vi "Main_Dev.vi"() -> ()   [LabVIEW 2020]
uses:
  <vilib>/Utility/file.llb/Read Delimited Spreadsheet (I64).vi
  <vilib>/Instr/_visa.llb/VISA Configure Serial Port (Serial Instr).vi
panel:
  out "Next MPH":u16
  out "Next Duration":u16
  out "Next Inc":u16
  out "PD READ 2":u8
  out "PD READ":u8
  out "INC READ":u8
  out "INC READ 2":u8
  out "MPH READ":u8
  out "MPH READ 2":u8
  out "dwell":u16[](array[numeric])
  out "incline":u16[](array[numeric])
  out "time":u16[](array[numeric])
  out "speed":u16[](array[numeric])
  out "selected path":path
  out "input lines":i32
  in  "TestScript":path=path "C:/LabView Computer Backup SEAL2788/DonP_TRM500/FootTimeInc.txt"
  out "refnum out":refnum<file>
  out "read buffer":string
  out "Target Changed":bool
  in  "stop":bool
  in  "Serial Port":refnum<visa-resource-name>="COM8"
  out "FootPath":path
  out "FootPathRef":refnum<file>
  out "stopping":bool
  out "Target MPH":u16 max=12 step=1
  out "step":i32
  out "ESTOP":bool
  out "ESTOP2":bool
  out "INC":u16 max=12 step=1
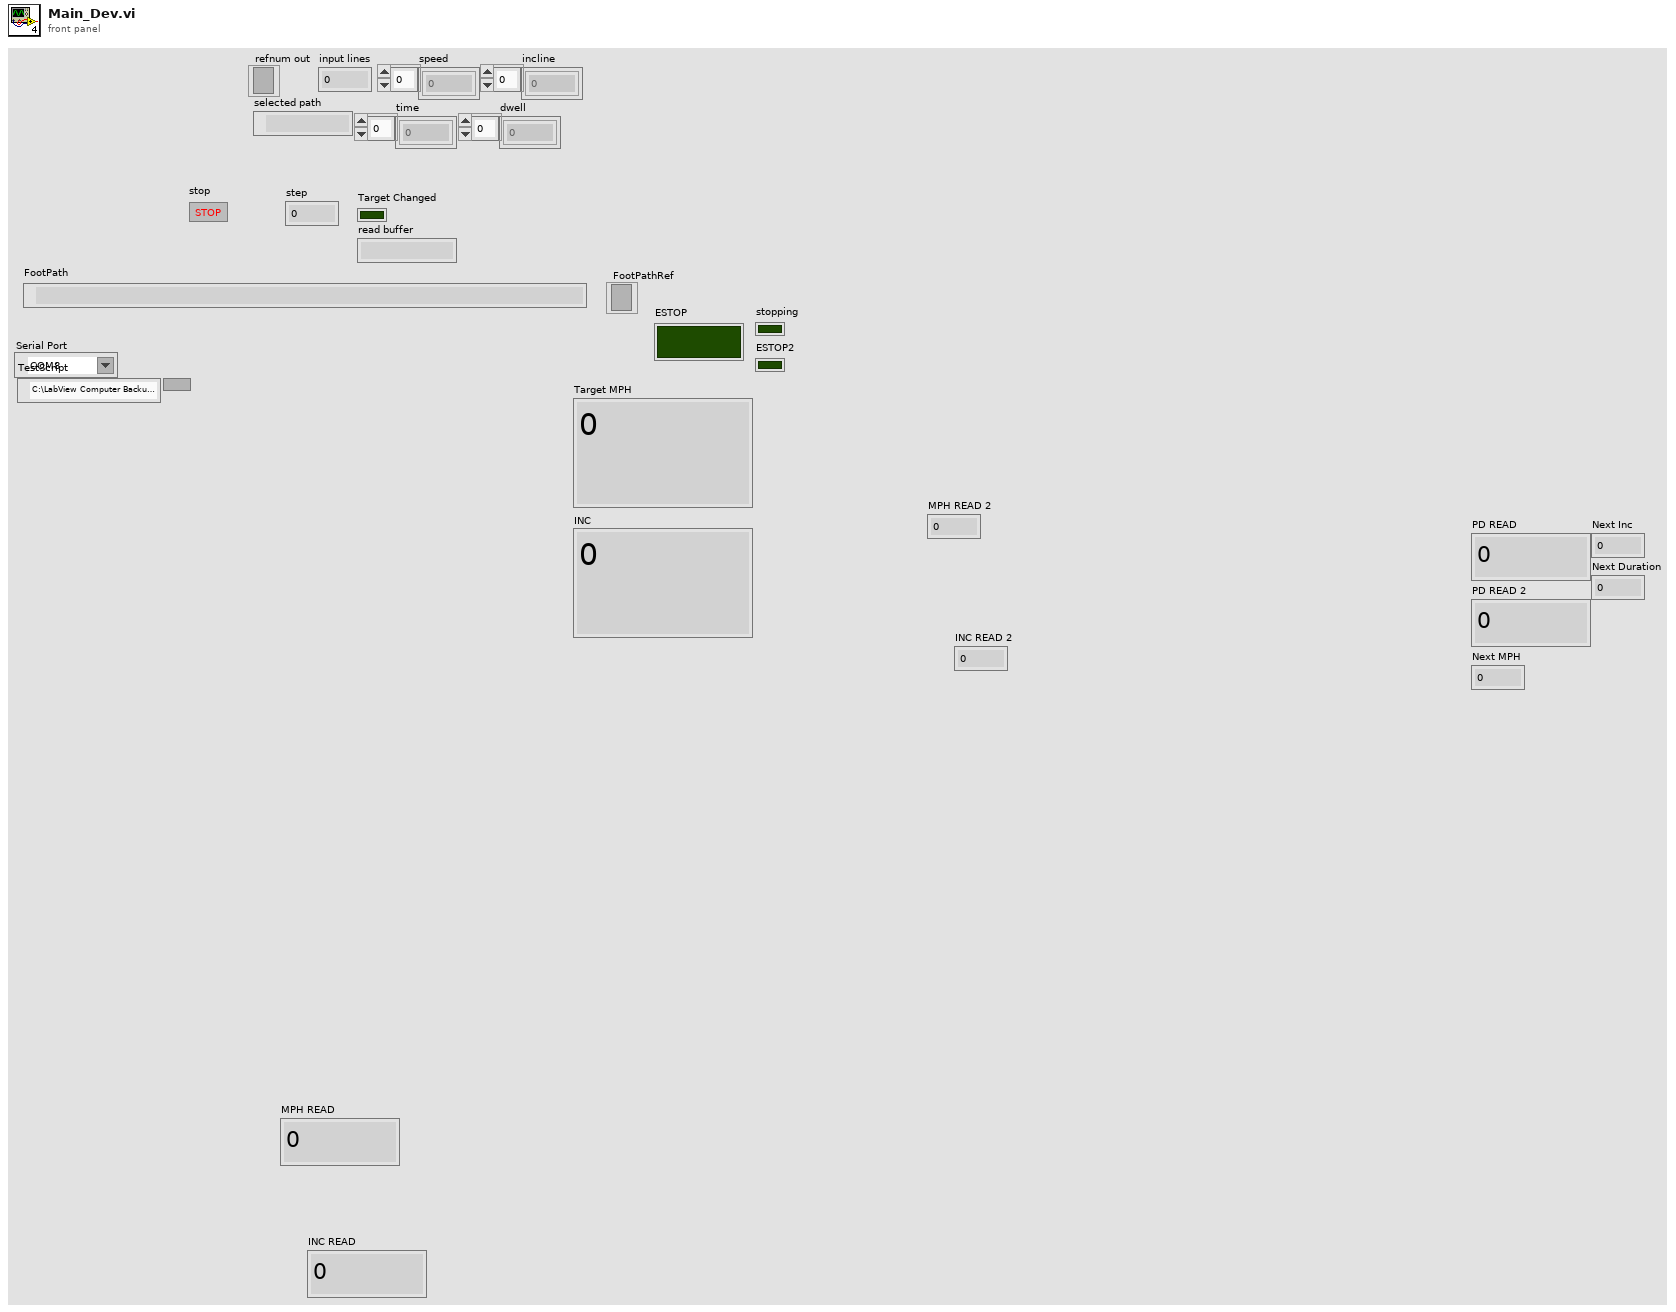
[diagram p1: front panel]
types:
  T1 = enum16{"Initialize", "SetTargets", "GetData", "CheckTiming", "CompressWave", "Dwell", "WaitforMPH", "ESTOP Wait", "ESTOP Resume"}
  T2 = cluster{"seconds since 1Jan1904":timestamp, "MPH":u8, "INC":u8}[]
  T3 = enum16{"Initialize", "SetMPH", "GetData", "CheckTiming", "CompressWave", "Dwell", "WaitforMPH", "ESTOP Wait", "ESTOP Resume"}
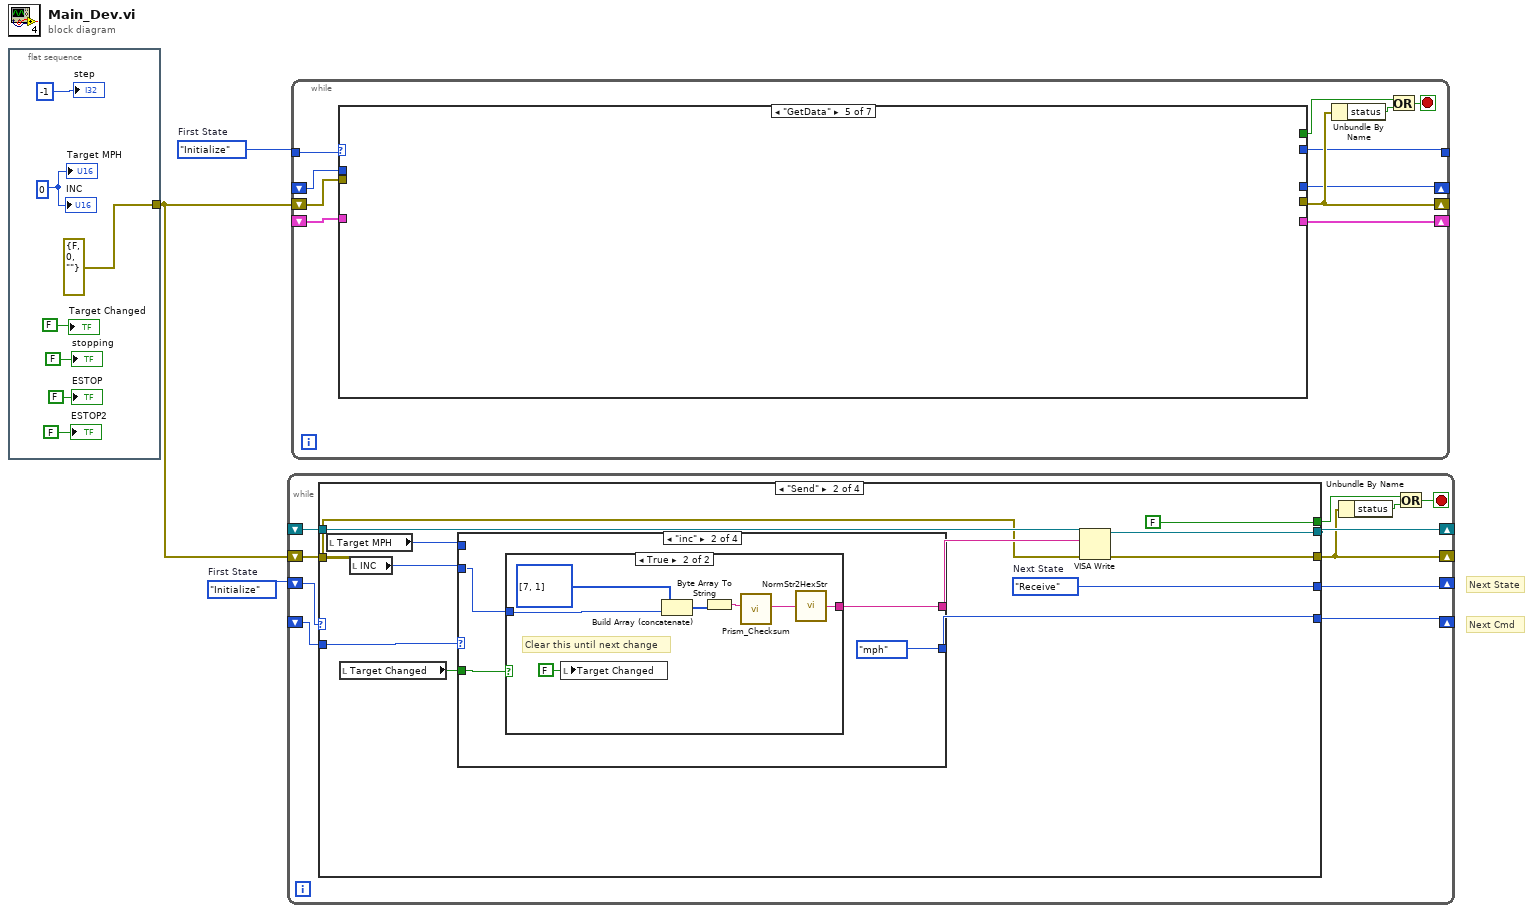
[diagram p0: block diagram]
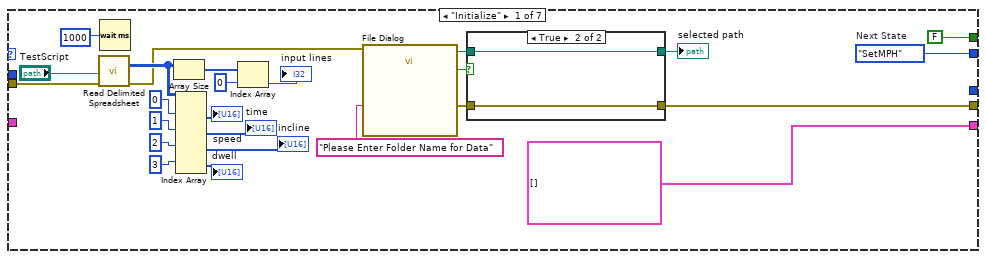
[diagram p2: hidden frame]
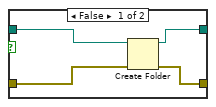
[diagram p3: hidden frame]
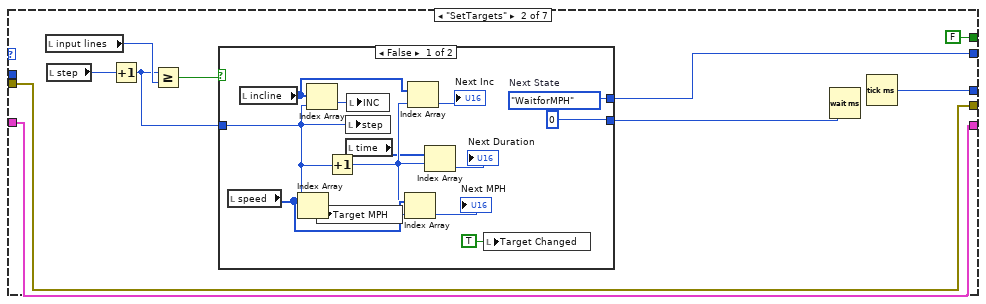
[diagram p4: hidden frame]
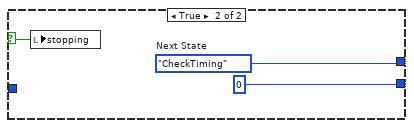
[diagram p5: hidden frame]
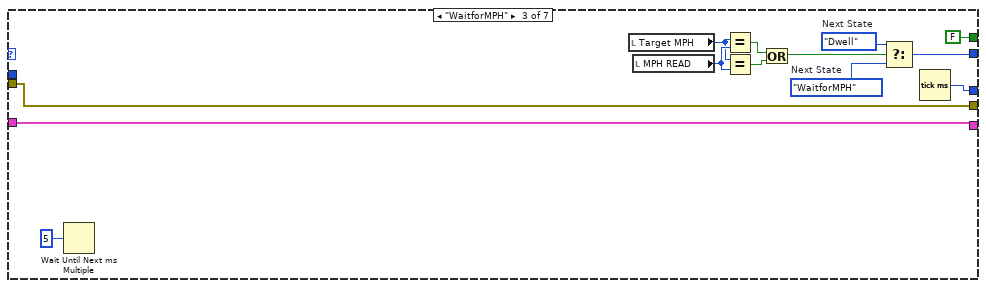
[diagram p6: hidden frame]
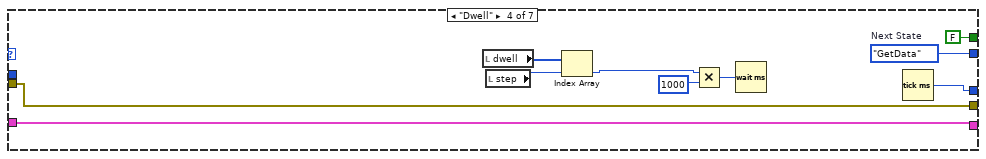
[diagram p7: hidden frame]
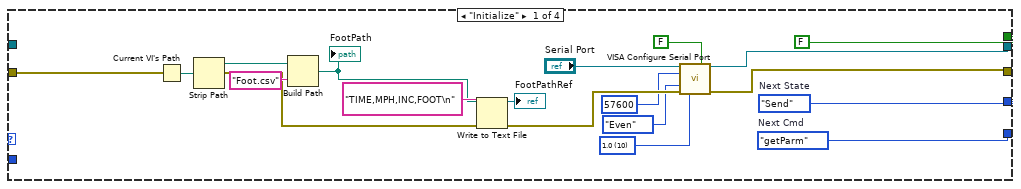
[diagram p10: hidden frame]
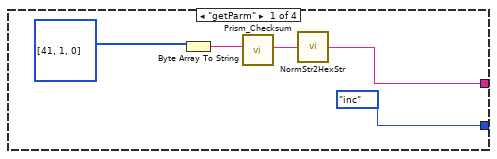
[diagram p11: hidden frame]
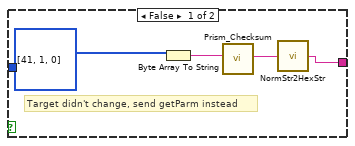
[diagram p12: hidden frame]
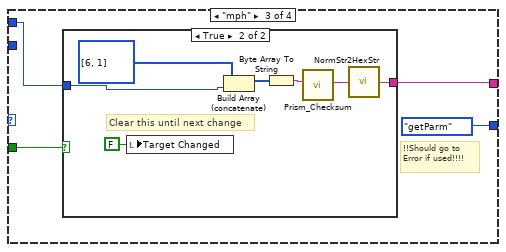
[diagram p13: hidden frame]
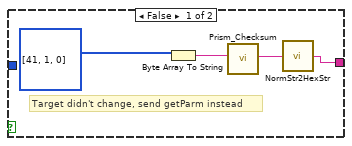
[diagram p14: hidden frame]
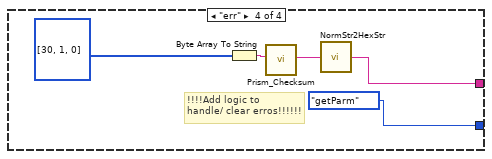
[diagram p15: hidden frame]
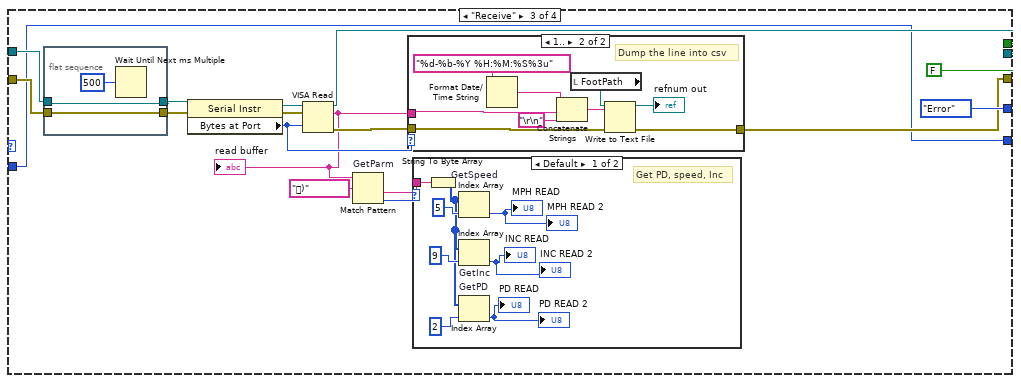
[diagram p16: hidden frame]
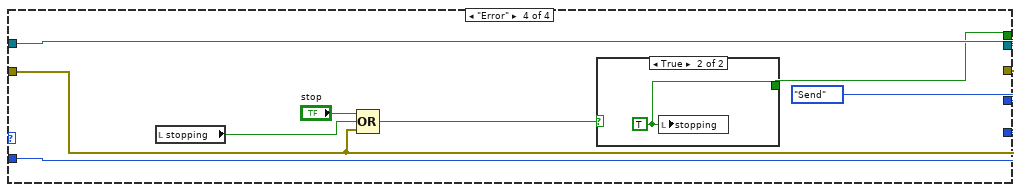
[diagram p19: hidden frame]
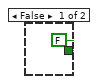
[diagram p20: hidden frame]
diagram:
  w1 = T1."Initialize"  # First State
  w3 = enum16{"Initialize", "Send", "Receive", "Error"}."Initialize"  # First State
  # "Next Cmd"
  # "Next State"
  n1 = flat-sequence {
    tunnel: [errorcluster {"status"=FALSE, "code"=0, "source"=""} ("error constant")] -> w2
    frame #0 {
      w4 = u16 0 ("MPH")
      "stopping" <- FALSE ("stopping")
      "Target MPH" <- w4
      "step" <- -1 ("step")
      "ESTOP" <- FALSE ("ESTOP")
      "ESTOP2" <- FALSE ("ESTOP2")
      "INC" <- w4
      "Target Changed" <- FALSE ("Value Changed")
    }
  }
  n2 = while {
    shift-right: [w13] -> _
    shift-left: w2 -> [w21]
    shift-right: [w18] -> _
    shift-left: _ -> [w20]
    shift-right: [w17] -> _
    shift-left: w3 -> [w19]
    shift-right: [w16] -> _
    shift-left: _ -> [w15]
    stop <- w12 stop-if-true
    n3 = case shown="\"Send\"" w19 {
      tunnel: w21 -> [w27 w42 w101 w131]
      tunnel: w20 -> [_ w49 w105 w135]
      tunnel: [w37 w51 w104 w135] -> w18
      tunnel: [w36 w50 w98 w131] -> w13
      tunnel: [w33 w45 enum16{"Initialize", "Send", "Receive", "Error"}."Error" enum16{"Initialize", "Send", "Receive", "Error"}."Send"] -> w17
      tunnel: [w35 w43 w92 w136] -> w16
      tunnel: w15 -> [_ w41 w92 w136]
      tunnel: [FALSE FALSE FALSE w130] -> w14
      frame "Initialize" {
        w22 = u16 10 items=["1.0"=10, "1.5"=15, "2.0"=20] ("stop bits (10: 1 bit)")
        w33 = enum16{"Initialize", "Send", "Receive", "Error"}."Send"  # Next State
        w35 = enum16{"getParm", "inc", "mph", "err"}."getParm"  # Next Cmd
        n4 = Current VI's Path() -> (path=w32:path)
        n5 = Strip Path(path=w32) -> (stripped path=w31:path)  [unwired: 1 out]
        n6 = Build Path(base path=w31, name or relative path="Foot.csv") -> (appended path=w28:path)
        "FootPath" <- w28
        n7 = Write to Text File(file (use dialog)=w28, text="TIME,MPH,INC,FOOT\n", error in=w27) -> (refnum out=→"FootPathRef":refnum<file>, error out=w26:errorcluster)  [unwired: 1 in, 1 out]
        n8 = call-poly "VISA Configure Serial Port"("VISA resource name"="Serial Port", "Enable Termination\nChar (T)"=FALSE ("Enable Termination\nChar (T)"), "baud rate (9600)"=u32 57600, "parity (0:none)"=enum16{"None", "Odd", "Even", "Mark", "Space"}."Even", "error in (no error)"=w26, "stop bits (10: 1 bit)"=w22) -> ("VISA resource name out"=w37:refnum<visa-resource-name>, "error out"=w36:errorcluster)  [unwired: 8 in]
      }
      frame "Send" {
        w45 = enum16{"Initialize", "Send", "Receive", "Error"}."Receive"  # Next State
        n9 = local read "Target MPH"() -> (w47:u16)
        n10 = local read "Target Changed"() -> (w40:bool)
        n11 = local read "INC"() -> (w46:u16)
        n12 = case shown="\"inc\"" w41 {
          tunnel: w47 -> [_ _ w72 _]
          tunnel: w46 -> [_ w59 _ _]
          tunnel: [w52 w58 w73 w88] -> w44
          tunnel: [enum16{"getParm", "inc", "mph", "err"}."inc" enum16{"getParm", "inc", "mph", "err"}."mph" enum16{"getParm", "inc", "mph", "err"}."getParm" enum16{"getParm", "inc", "mph", "err"}."getParm"] -> w43
          tunnel: w40 -> [_ w60 w75 _]
          frame "getParm" {
            n13 = Byte Array To String(unsigned byte array=u8[] [41, 1, 0]) -> (string=w54:string)
            n14 = call "Prism_Checksum.vi"("ID +DB+ Data"=w54) -> ("Full Cmd"=w53:string)  [unwired: 10 in]
            n15 = call "NormStr2HexStr.vi"("string"=w53) -> ("hex string"=w52:string)
          }
          frame "inc" {
            n16 = case shown="True" w60 {
              tunnel: w59 -> [_ w68]
              tunnel: [w61 w66] -> w58
              frame False {
                # "Target didn't change, send getParm instead"
                n17 = Byte Array To String(unsigned byte array=u8[] [41, 1, 0]) -> (string=w63:string)
                n18 = call "Prism_Checksum.vi"("ID +DB+ Data"=w63) -> ("Full Cmd"=w62:string)  [unwired: 10 in]
                n19 = call "NormStr2HexStr.vi"("string"=w62) -> ("hex string"=w61:string)
              }
              frame True {
                # "Clear this until next change"
                n20 = local write "Target Changed"(FALSE ("Value Changed")) -> ()
                n21 = Build Array (concatenate)(u8[] [7, 1] ("unsigned byte array"), w68) -> (w67:u16[])
                n22 = Byte Array To String(unsigned byte array=w67) -> (string=w70:string)
                n23 = call "Prism_Checksum.vi"("ID +DB+ Data"=w70) -> ("Full Cmd"=w71:string)  [unwired: 10 in]
                n24 = call "NormStr2HexStr.vi"("string"=w71) -> ("hex string"=w66:string)
              }
            }
          }
          frame "mph" {
            # "!!Should go to\nError if used!!!!"
            n25 = case shown="True" w75 {
              tunnel: [w76 w83] -> w73
              tunnel: w72 -> [_ w81]
              frame False {
                # "Target didn't change, send getParm instead"
                n26 = Byte Array To String(unsigned byte array=u8[] [41, 1, 0]) -> (string=w78:string)
                n27 = call "Prism_Checksum.vi"("ID +DB+ Data"=w78) -> ("Full Cmd"=w77:string)  [unwired: 10 in]
                n28 = call "NormStr2HexStr.vi"("string"=w77) -> ("hex string"=w76:string)
              }
              frame True {
                # "Clear this until next change"
                n29 = local write "Target Changed"(FALSE ("Value Changed")) -> ()
                n30 = Build Array (concatenate)(u8[] [6, 1] ("unsigned byte array"), w81) -> (w82:u16[])
                n31 = Byte Array To String(unsigned byte array=w82) -> (string=w85:string)
                n32 = call "Prism_Checksum.vi"("ID +DB+ Data"=w85) -> ("Full Cmd"=w86:string)  [unwired: 10 in]
                n33 = call "NormStr2HexStr.vi"("string"=w86) -> ("hex string"=w83:string)
              }
            }
          }
          frame "err" {
            # "!!!!Add logic to\nhandle/ clear erros!!!!!!"
            n34 = Byte Array To String(unsigned byte array=u8[] [30, 1, 0]) -> (string=w90:string)
            n35 = call "Prism_Checksum.vi"("ID +DB+ Data"=w90) -> ("Full Cmd"=w91:string)  [unwired: 10 in]
            n36 = call "NormStr2HexStr.vi"("string"=w91) -> ("hex string"=w88:string)
          }
        }
        n37 = VISA Write(VISA resource name=w49, write buffer=w44, error in (no error)=w42) -> (VISA resource name out=w51:refnum<visa-resource-name>, error out=w50:errorcluster)  [unwired: 1 out]
      }
      frame "Receive" {
        n38 = flat-sequence {
          tunnel: w105 -> [w128]
          tunnel: [w128] -> w108
          tunnel: w101 -> [w127]
          tunnel: [w127] -> w100
          frame #0 {
            n39 = Wait Until Next ms Multiple(millisecond multiple=u32 500) -> ()  [unwired: 1 out]
          }
        }
        n40 = property class="Serial Instr"(reference=w108, error in=w100) -> (reference out=w106:refnum<visa-resource-name>, error out=w107:errorcluster, "Bytes at Port"=w99:u32)
        n41 = VISA Read(VISA resource name=w106, byte count=w99, error in (no error)=w107) -> (VISA resource name out=w104:refnum<visa-resource-name>, read buffer=w93:string, error out=w97:errorcluster)  [unwired: 1 out]
        "read buffer" <- w93
        n42 = Match Pattern "GetParm"(string=w93, regular expression="ޭ)") -> (after substring=w95:string, offset past match=w96:i32)  [unwired: 1 in, 2 out]
        n43 = case shown="1.." w99 {
          tunnel: w93 -> [_ w120]
          tunnel: [w117 w119] -> w98
          tunnel: w97 -> [w117 w118]
          frame 0 {
          }
          frame 1.. {
            # "Dump the line into csv"
            n44 = Format Date/Time String(time format string (%c)="%d-%b-%Y %H:%M:%S%3u") -> (date/time string=w126:string)  [unwired: 2 in]
            n45 = Concatenate Strings(w126, w120, "\r\n") -> (w123:string)
            n46 = local read "FootPath"() -> (w124:path)
            n47 = Write to Text File(file (use dialog)=w124, text=w123, error in=w118) -> (refnum out=→"refnum out":refnum<file>, error out=w119:errorcluster)  [unwired: 1 in, 1 out]
          }
        }
        n48 = case shown="Default" w96 {
          tunnel: w95 -> [w116 _]
          frame Default {
            # "Get PD, speed, Inc"
            n49 = String To Byte Array(string=w116) -> (unsigned byte array=w110:u8[])
            n50 = Index Array "GetSpeed"(array=w110, index=5) -> (element=→"MPH READ" →"MPH READ 2":u8)
            n51 = Index Array "GetInc"(array=w110, index=9) -> (element=→"INC READ" →"INC READ 2":u8)
            n52 = Index Array "GetPD"(array=w110, index=2) -> (element=→"PD READ" →"PD READ 2":u8)
          }
          frame -1 {
          }
        }
      }
      frame "Error" {
        n53 = local read "stopping"() -> (w132:bool)
        n54 = Compound Arithmetic op=OR("stop", w132, w131) -> (w134:bool)
        n55 = case shown="True" w134 {
          tunnel: [FALSE w139] -> w130
          frame False {
          }
          frame True {
            w139 = TRUE ("stopping")
            n56 = local write "stopping"(w139) -> ()
          }
        }
      }
    }
    n57 = Unbundle By Name(w13) -> ("status"=w11:bool)
    n58 = Or(x=w14, y=w11) -> (x .or. y?=w12:bool)
  }
  n59 = while {
    shift-right: [w146] -> _
    shift-left: w2 -> [w150]
    shift-right: [w145] -> _
    shift-left: _ -> [w144]
    tunnel: w1 -> [w142]
    tunnel: [w143] -> _
    shift-right: [w141] -> _
    shift-left: _ -> [w140]
    stop <- w148 stop-if-true
    n60 = case shown="\"GetData\"" w142 {
      tunnel: w150 -> [w173 w186 w219 w226 _ _ _]
      tunnel: [FALSE FALSE FALSE FALSE _ _ _] -> w147
      tunnel: [w157 w186 w219 w226 _ _ _] -> w146
      tunnel: [T2 [] w185 w218 w227 _ _ _] -> w145
      tunnel: w144 -> [_ w185 w218 w227 _ _ _]
      tunnel: [w155 w188 w213 w223 _ _ _] -> w143
      tunnel: [_ w183 w216 w222 _ _ _] -> w141
      tunnel: w140 -> [_ _ _ _ _ _ _]
      frame "Initialize" {
        w155 = T3."SetMPH"  # Next State
        n61 = call-poly <vilib>:"Read Delimited Spreadsheet.vi"("file path (dialog if empty)"="TestScript", "error in (no error)"=w173) -> ("all rows"=w169:i64[][], "error out"=w164:errorcluster)  [unwired: 8 in, 4 out]
        n62 = Wait (ms)(milliseconds to wait=u32 1000) -> ()  [unwired: 1 out]
        n63 = Array Size(array=w169) -> (size(s)=w171:i32[])
        n64 = Index Array(array=w169, index (row) #1=0 ("index"), index (row) #2=1 ("index (col)"), index (row) #3=2 ("index (col)"), index (row) #4=3 ("index (col)")) -> (element #1=→"speed":i64[], element #2=→"time":i64[], element #3=→"incline":i64[], element #4=→"dwell":i64[])  [unwired: 4 in]
        n65 = Index Array(array=w171, index=0) -> (element=→"input lines":i32)
        n66 = call "File Dialog"("prompt"="Please Enter Folder Name for Data", "error in"=w164) -> ("selected path"=w162:path, "exists"=w161:bool, "error out"=w160:errorcluster)  [unwired: 10 in, 1 out]
        n67 = case shown="True" w161 {
          tunnel: w160 -> [w179 w181]
          tunnel: w162 -> [w178 w180]
          tunnel: [w177 w181] -> w157
          tunnel: [w176 w180] -> w159
          frame False {
            n68 = Create Folder(path (use dialog)=w178, error in=w179) -> (created path=w176:path, error out=w177:errorcluster)  [unwired: 1 in, 1 out]
          }
          frame True {
          }
        }
        "selected path" <- w159
      }
      frame "SetTargets" {
        n69 = local read "input lines"() -> (w190:i32)
        n70 = local read "step"() -> (w191:i32)
        n71 = Increment(x=w191) -> (x+1=w182:i32)
        n72 = Greater Or Equal?(x=w182, y=w190) -> (x >= y?=w189:bool)
        n73 = case shown="False" w189 {
          selector: w189 -> [_ w207]
          tunnel: [w204 w206] -> w188
          tunnel: [u32 0 ("milliseconds to wait") u32 0 ("milliseconds to wait")] -> w187
          tunnel: w182 -> [w201 _]
          frame False {
            w204 = T1."WaitforMPH"  # Next State
            n74 = local read "speed"() -> (w200:u16[])
            n75 = local read "incline"() -> (w199:u16[])
            n76 = Index Array(array=w200, index=w201) -> (element=w203:u16)
            n77 = Index Array(array=w199, index=w201) -> (element=w202:u16)
            n78 = local write "Target MPH"(w203) -> ()
            n79 = Increment(x=w201) -> (x+1=w198:i32)
            n80 = local write "step"(w201) -> ()
            n81 = local read "time"() -> (w197:u16[])
            n82 = local write "INC"(w202) -> ()
            n83 = Index Array(array=w200, index=w198) -> (element=→"Next MPH":u16)
            n84 = Index Array(array=w199, index=w198) -> (element=→"Next Inc":u16)
            n85 = Index Array(array=w197, index=w198) -> (element=→"Next Duration":u16)
            n86 = local write "Target Changed"(TRUE ("Value Changed")) -> ()
          }
          frame True {
            w206 = T1."CheckTiming"  # Next State
            n87 = local write "stopping"(w207) -> ()
          }
        }
        n88 = Wait (ms)(milliseconds to wait=w187) -> ()  [unwired: 1 out]
        n89 = Tick Count (ms)() -> (millisecond timer value=w183:u32)
      }
      frame "WaitforMPH" {
        w215 = T1."Dwell"  # Next State
        w214 = T1."WaitforMPH"  # Next State
        n90 = Wait Until Next ms Multiple(millisecond multiple=u32 5) -> ()  [unwired: 1 out]
        n91 = local read "Target MPH"() -> (w208:u16)
        n92 = local read "MPH READ"() -> (w209:u8)
        n93 = Equal?(x=w208, y=w209) -> (x = y?=w211:bool)
        n94 = Equal?(x=w208, y=w209) -> (x = y?=w210:bool)
        n95 = Or(x=w211, y=w210) -> (x .or. y?=w212:bool)
        n96 = Select(t=w215, s=w212, f=w214) -> (s? t:f=w213:T1)
        n97 = Tick Count (ms)() -> (millisecond timer value=w216:u32)
      }
      frame "Dwell" {
        w223 = T1."GetData"  # Next State
        n98 = local read "dwell"() -> (w224:u16[])
        n99 = local read "step"() -> (w225:i32)
        n100 = Index Array(array=w224, index=w225) -> (element=w230:u16)
        n101 = Multiply(x=w230, y=u16 1000) -> (x*y=w228:u16)
        n102 = Wait (ms)(milliseconds to wait=w228) -> ()  [unwired: 1 out]
        n103 = Tick Count (ms)() -> (millisecond timer value=w222:u32)
      }
      frame "GetData" {
      }
      frame "CheckTiming" {
      }
      frame "CompressWave" {
      }
    }
    n104 = Unbundle By Name(w146) -> ("status"=w149:bool)
    n105 = Or(x=w147, y=w149) -> (x .or. y?=w148:bool)
  }
